vi "TMC_Split_Cluster.vi"(0 "TMC Cluster":T3) -> (1 "TMC-Status":T1, 4 "TMC-Control":T2)   [LabVIEW 2019]
uses:
  Torque_TMC/TMCCluster.ctl
  Torque_TMC/TMC_Control.ctl
  Torque_TMC/TMC_Status.ctl
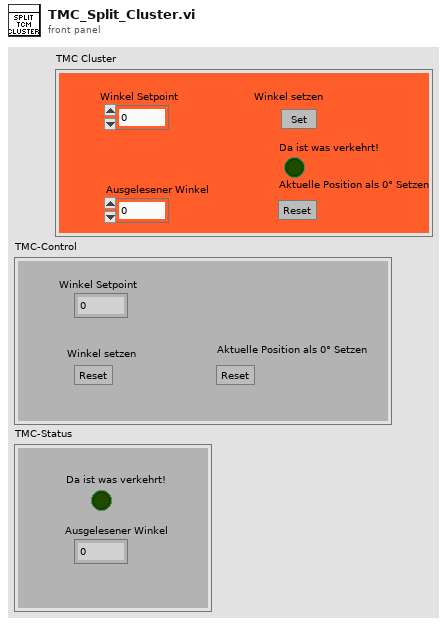
[diagram p1: front panel]
types:
  T1 = typedef "TMC_Status.ctl" = cluster{"Ausgelesener Winkel":dbl, "Da ist was verkehrt!":bool}
  T2 = typedef "TMC_Control.ctl" = cluster{"Winkel Setpoint":dbl, "Aktuelle Position als 0° Setzen":bool, "Winkel setzen":bool}
  T3 = typedef "TMCCluster.ctl" = cluster{"Winkel Setpoint":dbl, "Ausgelesener Winkel":dbl, "Aktuelle Position als 0° Setzen":bool, "Da ist was verkehrt!":bool, "Winkel setzen":bool}
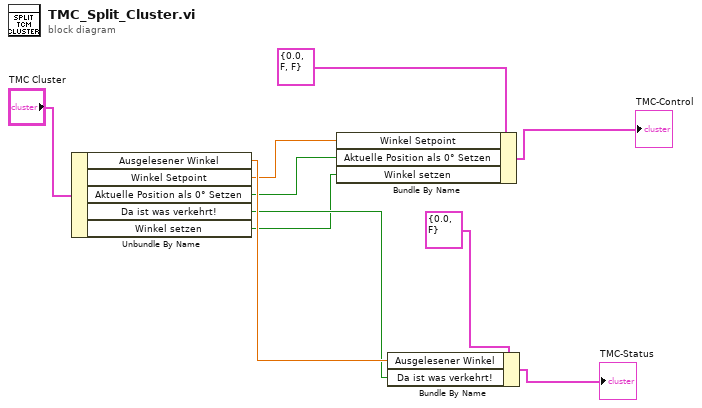
[diagram p0: block diagram]
diagram:
  n1 = Unbundle By Name("TMC Cluster") -> ("Ausgelesener Winkel"=w7:dbl, "Winkel Setpoint"=w1:dbl, "Aktuelle Position als 0° Setzen"=w4:bool, "Da ist was verkehrt!"=w6:bool, "Winkel setzen"=w2:bool)
  n2 = Bundle By Name(cluster=T2 {"Winkel Setpoint"=0.0, "Aktuelle Position als 0° Setzen"=FALSE, "Winkel setzen"=FALSE} ("TMC-Control"), "Winkel Setpoint"=w1, "Aktuelle Position als 0° Setzen"=w4, "Winkel setzen"=w2) -> (→"TMC-Control":T2)
  n3 = Bundle By Name(cluster=T1 {"Ausgelesener Winkel"=0.0, "Da ist was verkehrt!"=FALSE} ("TMC-Status"), "Ausgelesener Winkel"=w7, "Da ist was verkehrt!"=w6) -> (→"TMC-Status":T1)
